vi "Vision Processing.vi"(8 "error in (no error)":errorcluster, 11 "Image Size":T2=enum."320x240") -> ()   [LabVIEW 2016]
uses:
  Program Files (x86)/National Instruments/LabVIEW 2016/examples/FRC/roboRIO/Vision/2017 Vision Example/Vision Support Code/Camera Types.ctl
  <vilib>/Rock Robotics/WPI/Camera/WPI_CameraImageSize.ctl
  <vilib>/Rock Robotics/WPI/Camera/WPI_CameraFrameRate.ctl
  <vilib>/Rock Robotics/WPI/Camera/WPI_CameraWhite Balance Values.ctl
  <vilib>/Rock Robotics/WPI/Camera/WPI_CameraExposure Values.ctl
  Robot Global Data.vi
  <vilib>/Rock Robotics/Network Tables/NT Write Number.vi
  <vilib>/vision/NI_Vision_Development_Module.lvlib
panel:
  in  "Frame Rate (fps)":T1=5
  in  "No vis code espos %":dbl format="%#_13g"
  out "error out":errorcluster
  in  "Size Limit %":dbl=0.02 format="%#_13g"
  in  "Ideal Target Height (in)":dbl=10.0
  out "loop ms":u32
  out "Calibration error":errorcluster
  in  "Display Original":bool
  in  "Display Mask":bool
  in  "Line Border":cluster{"Top":dbl, "Bottom":dbl}={"Top"=6.0, "Bottom"=1.0}
  in  "Use Calibration":bool
  out "Instructions:":string="Use Source to load image files from a directory, or use a USB or IP camera connected to your laptop. Use Camera Settings 1 and 2 to achieve a dark image with bright and colorful stripes.\nLED Color can encoded as HSL or related color modes. Calibrate to the same color as the strips being reflected to the camera.\nClick and draw a line in Original Image to auto-calibrate the LED Color. You may want to widen and tweak Sat and Val by hand.\nThe Annotate button affects drawing a rectangle around the stripes and labeling it with a distance in ft. Distance relies on knowing the Camera Type and lens calibration (it looks up the lens view angle).\n\nAdjust Score Cutoff to make the code more or less picky. If the color is not very unique, you may need to increase the number of particles considered. The diagram uses a Size Limit to ignore colored things that are too small. You may need to adjust it if you are targetting from far away.\n\nResults give you the distance to the target, the center and box in a normalized (-1 to 1) and pixel coordinates.\n\nBe sure to read about setting camera exposure and brightness to help simplify your image and acquire color saturated images.\n\nThere are lots of comments on the diagram to explain the code."
  in  "Color Mode":u16(ring)=3 items=["RGB", "HSL", "HSV", "HSI"]
  in  "Particles":dbl=5.0
  in  "Score Cutoff %":dbl=70.0
  in  "Camera Type":T3=enum."MS HD3000 640x480"
  out "Results":T4 {"Score" format="%#_3g"; "Pixels"."Rectangle"."Numeric 5" format="%#_3g"; "Pixels"."Rectangle"."Numeric 3" format="%#_3g"; "Pixels"."Rectangle"."Numeric 2" format="%#_3g"; "Pixels"."Rectangle"."Numeric" format="%#_3g"; "Normalized"."Rectangle"."Numeric 5" format="%#_2g"; "Normalized"."Rectangle"."Numeric 3" format="%#_2g"; "Normalized"."Rectangle"."Numeric 2" format="%#_2g"; "Normalized"."Rectangle"."Numeric" format="%#_2g"; "Normalized"."Center"."?" format="%#_3g"; "Normalized"."Center"."?" format="%#_3g"; "Distance (ft)" format="%#_3g"}
  out "Qualified Particles":i32
  in  "LED Color":T5={"Hue"={92.0569503435165, 129.13526899568942}, "Sat"={176.07142857142858, 255.0}, "Val"={40.53571428571429, 255.0}} {"Hue" scale=0.0..255.0 scale format="%#_3g"}
  out "Mask":T6(plugin-control)
  out "Original Image":T6(plugin-control)
  # "Legend:\n    Rectangle\n       Green - Good target, distance ft\n       Red - Bad target\n    Orange Text - Score in %"
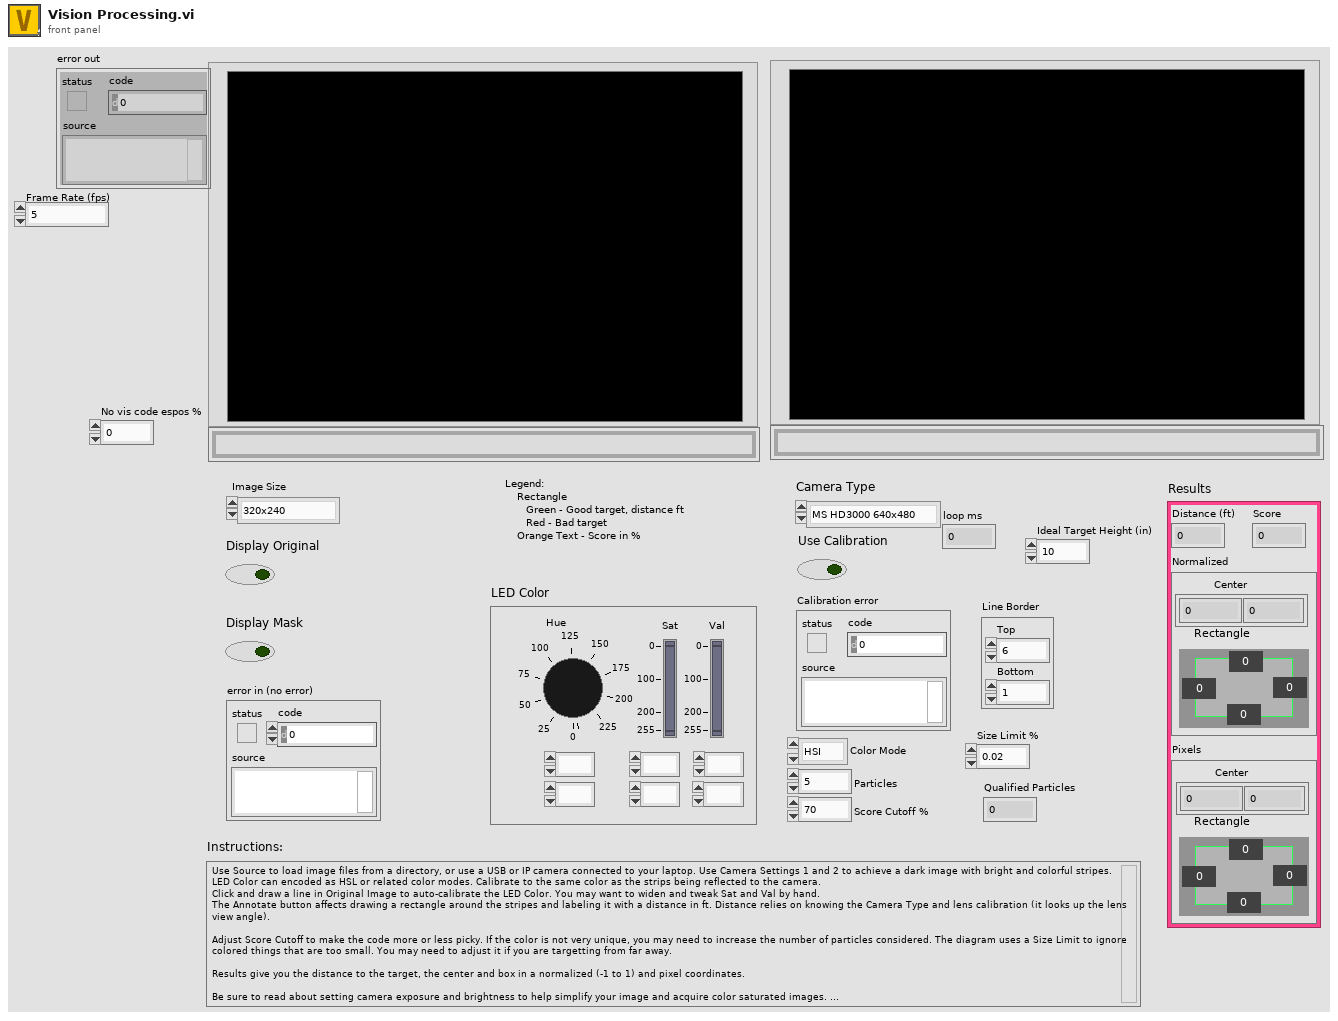
[diagram p1: front panel]
types:
  T1 = typedef "WPI_CameraFrameRate.ctl" = u32
  T2 = typedef "WPI_CameraImageSize.ctl" = enum16{"640x480", "320x240", "160x120", "Custom"}
  T3 = typedef "Camera Types.ctl" = enum16{"206", "1011", "1013", "MS HD3000 square", "MS HD3000 640x480"}
  T4 = cluster{"Distance (ft)":dbl, "Score":dbl, "Normalized":cluster{"Center":cluster{dbl, dbl}, "Rectangle":cluster{"Numeric":dbl, "Numeric 2":dbl, "Numeric 3":dbl, "Numeric 5":dbl}}, "Pixels":cluster{"Center":cluster{dbl, dbl}, "Rectangle":cluster{"Numeric":dbl, "Numeric 2":dbl, "Numeric 3":dbl, "Numeric 5":dbl}}}
  T5 = cluster{"Hue":cluster{dbl, dbl}, "Sat":cluster{dbl, dbl}, "Val":cluster{dbl, dbl}}
  T6 = typedef "IMAQ Image.ctl" = refnum<image>
  T7 = typedef "WPI_CameraWhite Balance Values.ctl" = enum16{"Auto", "Fixed indoor", "Fixed outdoor 1", "Fixed outdoor 2", "Fixed fluorescent 1", "Fixed fluorescent 2", "Hold current", "Custom"}
  T8 = typedef "Particle Parameters" = i32
  T9 = typedef "Image Type" = u32
  T10 = typedef "WPI_CameraDevRef.ctl" = cluster{"Camera Address":string, "CameraStatus":errorcluster}
  T11 = typedef "WPI_CameraExposure Values.ctl" = enum16{"Auto", "Flicker-free 50 Hz", "Flicker-free 60 Hz", "Hold current", "Custom"}
  T12 = cluster{"Left":dbl, "Top":dbl, "Right":dbl, "Bottom":dbl}
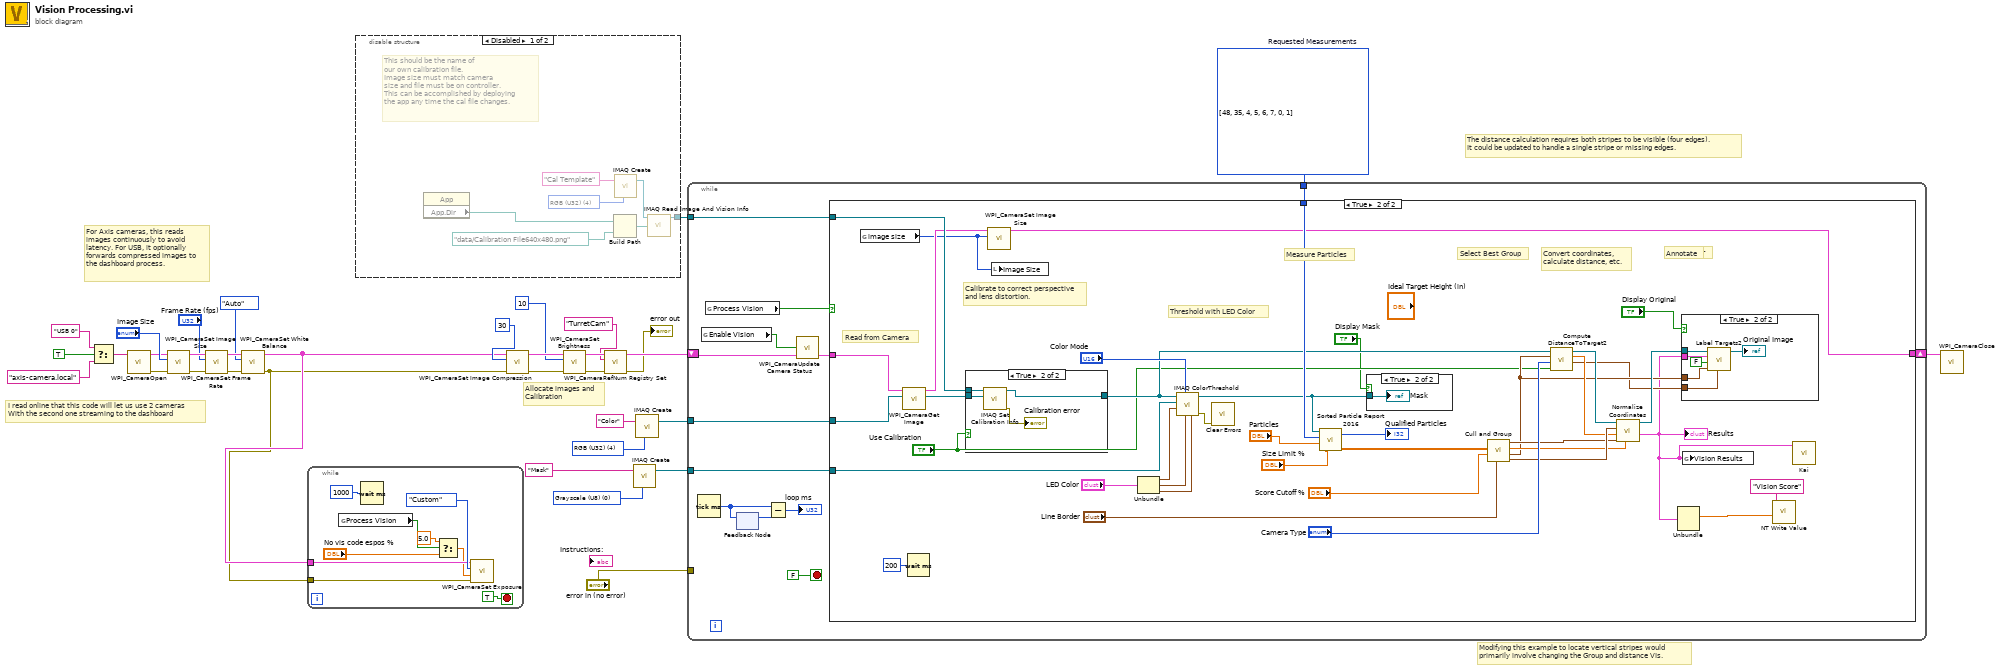
[diagram p0: block diagram]
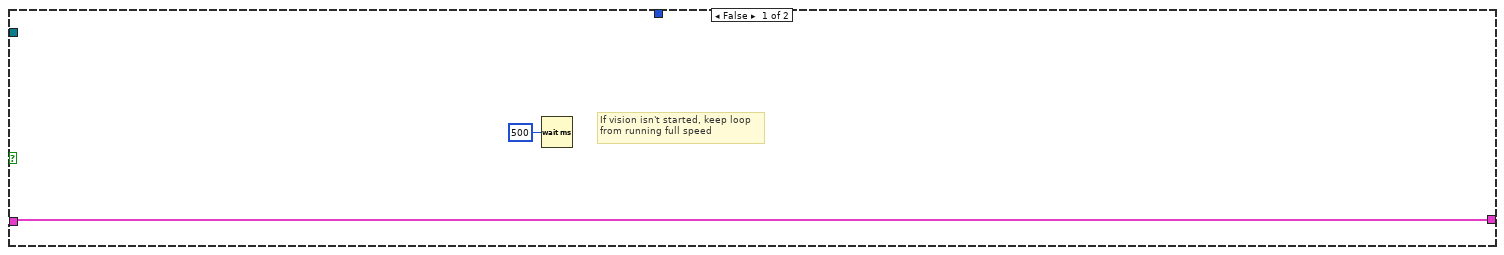
[diagram p3: hidden frame]
diagram:
  w29 = T8[] [48, 35, 4, 5, 6, 7, 0, 1] items=["Center of Mass X", "Center of Mass Y", "First Pixel X", "First Pixel Y", "Bounding Rect Left", "Bounding Rect Top", "Bounding Rect Right", "Bounding Rect Bottom", "Max Feret Diameter Start X", "Max Feret Diameter Start Y", "Max Feret Diameter End X", "Max Feret Diameter End Y", "Max Horiz. Segment Length Left", "Max Horiz. Segment Length Right", "Max Horiz. Segment Length Row", "-", "Bounding Rect Width", "Bounding Rect Height", "Bounding Rect Diagonal", "Perimeter", "Convex Hull Perimeter", "Holes' Perimeter", "Max Feret Diameter", "Equivalent Ellipse Major Axis", "Equivalent Ellipse Minor Axis", "Equivalent Ellipse Minor Axis (Feret)", "Equivalent Rect Long Side", "Equivalent Rect Short Side", "Equivalent Rect Diagonal", "Equivalent Rect Short Side (Feret)", "Average Horiz. Segment Length", "Average Vert. Segment Length", "Hydraulic Radius", "Waddel Disk Diameter", "-", "Area", "Holes' Area", "Particle & Holes' Area", "Convex Hull Area", "Image Area", "-", "Number of Holes", "Number of Horiz. Segments", "Number of Vert. Segments", "-", "Orientation", "Max Feret Diameter Orientation", "-", "% Area/Image Area", "% Area/(Particle & Holes' Area)", "Ratio of Equivalent Ellipse Axes", "Ratio of Equivalent Rect Sides", "-", "Elongation Factor", "Compactness Factor", "Heywood Circularity Factor", "Type Factor", "-", "Sum X", "Sum Y", "Sum XX", "Sum XY", "Sum YY", "Sum XXX", "Sum XXY", "Sum XYY", "Sum YYY", "-", "Moment of Inertia XX", "Moment of Inertia XY", "Moment of Inertia YY", "Moment of Inertia XXX", "Moment of Inertia XXY", "Moment of Inertia XYY", "Moment of Inertia YYY", "Norm. Moment of Inertia XX", "Norm. Moment of Inertia XY", "Norm. Moment of Inertia YY", "Norm. Moment of Inertia XXX", "Norm. Moment of Inertia XXY", "Norm. Moment of Inertia XYY", "Norm. Moment of Inertia YYY", "Hu Moment 1", "Hu Moment 2", "Hu Moment 3", "Hu Moment 4", "Hu Moment 5", "Hu Moment 6", "Hu Moment 7"]  # Requested Measurements
  w32 = T9 0 items=["Grayscale (U8)", "Grayscale (I16)", "Grayscale (SGL)", "Complex (CSG)", "RGB (U32)", "HSL (U32)", "RGB (U64)", "Grayscale (U16)"] ("Image Type")
  w33 = T9 4 items=["Grayscale (U8)", "Grayscale (I16)", "Grayscale (SGL)", "Complex (CSG)", "RGB (U32)", "HSL (U32)", "RGB (U64)", "Grayscale (U16)"] ("Image Type")
  # "I read online that this code will let us use 2 cameras\nWith the second one streaming to the dashboard"
  # "For Axis cameras, this reads\nimages continuously to avoid\nlatency. For USB, it optionally\nforwards compressed images to\nthe dashboard process."
  # "Modifying this example to locate vertical stripes would\nprimarily involve changing the Group and distance VIs."
  # "The distance calculation requires both stripes to be visible (four edges).\nIt could be updated to handle a single stripe or missing edges."
  # "Allocate images and\nCalibration"
  n1 = Select(t="USB 0" ("format string"), s=TRUE ("dot notation? (F)"), f="axis-camera.local" ("format string")) -> (s? t:f=w8:string)
  n2 = call <vilib>:"WPI_CameraOpen.vi"("Camera Address"=w8) -> ("error out"=w17:errorcluster, "CameraDevRef"=w18:T10)  [unwired: 2 in, 7 out]
  n3 = call <vilib>:"WPI_CameraSet Image Size.vi"("error in (no error)"=w17, "Image Size"="Image Size", "CameraDevRef"=w18) -> ("error out"=w16:errorcluster, "CameraDevRef Out"=w19:T10)  [unwired: 1 in, 6 out]
  n4 = call <vilib>:"WPI_CameraSet Frame Rate.vi"("error in (no error)"=w16, "Frame Rate (fps)"="Frame Rate (fps)", "CameraDevRef"=w19) -> ("error out"=w15:errorcluster, "CameraDevRef Out"=w20:T10)  [unwired: 7 out]
  n5 = call <vilib>:"WPI_CameraSet White Balance.vi"("error in (no error)"=w15, "White Balance"=WPI_CameraWhite_Balance_Values."Auto", "CameraDevRef"=w20) -> ("error out"=w1:errorcluster, "CameraDevRef Out"=w2:T10)  [unwired: 1 in, 6 out]
  n6 = while {
    tunnel: w2 -> [w42]
    tunnel: w1 -> [w41]
    stop <- TRUE stop-if-true
    n7 = global read "Robot Global Data.vi" "Process Vision"() -> (w38:bool)
    n8 = Wait (ms)(milliseconds to wait=u32 1000) -> ()  [unwired: 1 out]
    n9 = Select(t=5.0 ("Exposure (%)"), s=w38, f="No vis code espos %") -> (s? t:f=w35:dbl)
    n10 = call <vilib>:"WPI_CameraSet Exposure.vi"("error in (no error)"=w41, "Exposure (%)"=w35, "Exposure"=WPI_CameraExposure_Values."Custom", "CameraDevRef"=w42) -> ()  [unwired: 8 out]
  }
  n11 = disable-structure shown="Disabled" {
    disable-tunnel: [w47 _] -> w27
    frame Disabled {
      w50 = T9 4 items=["Grayscale (U8)", "Grayscale (I16)", "Grayscale (SGL)", "Complex (CSG)", "RGB (U32)", "HSL (U32)", "RGB (U64)", "Grayscale (U16)"] ("Image Type")
      # "This should be the name of \nour own calibration file.\nImage size must match camera\nsize and file must be on controller.\nThis can be accomplished by deploying\nthe app any time the cal file changes."
      n12 = property class="App"() -> ("App.Dir"=w44:path)  [unwired: 2 in, 2 out]
      n13 = Build Path(base path=w44, name or relative path=path "data/Calibration File640x480.png" ("Folder Location")) -> (appended path=w46:path)
      n14 = call "IMAQ Create"("Image Name"="Cal Template", "Image Type"=w50) -> ("New Image"=w48:T6)  [unwired: 2 in, 2 out]
      n15 = call "IMAQ Read Image And Vision Info"("File Path"=w46, "Image"=w48) -> ("Image Out"=w47:T6)  [unwired: 7 in, 2 out]
    }
    frame Enabled {
    }
  }
  n16 = call <vilib>:"WPI_CameraSet Image Compression.vi"("error in (no error)"=w1, "Compression"=30, "CameraDevRef"=w2) -> ("error out"=w14:errorcluster, "CameraDevRef Out"=w21:T10)  [unwired: 7 out]
  n17 = call <vilib>:"WPI_CameraSet Brightness.vi"("error in (no error)"=w14, "Brightness"=10, "CameraDevRef"=w21) -> ("error out"=w13:errorcluster, "CameraDevRef Out"=w26:T10)  [unwired: 7 out]
  n18 = call <vilib>:"WPI_CameraRefNum Registry Set.vi"("error in (no error)"=w13, "refnum name"="TurretCam", "CameraDevRef"=w26) -> ("error out"=→"error out":errorcluster, "CameraDevRef"=w7:T10)  [unwired: 1 in, 6 out]
  n19 = call "IMAQ Create"("Image Name"="Mask", "Image Type"=w32) -> ("New Image"=w30:T6)  [unwired: 2 in, 2 out]
  n20 = call "IMAQ Create"("Image Name"="Color", "Image Type"=w33) -> ("New Image"=w28:T6)  [unwired: 2 in, 2 out]
  n21 = while {
    tunnel: w28 -> [w59]
    tunnel: w30 -> [w62]
    tunnel: w29 -> [w61]
    tunnel: w27 -> [w60]
    shift-right: [w58] -> w6
    shift-left: w7 -> [w57]
    tunnel: "error in (no error)" -> [_]
    stop <- FALSE stop-if-true
    n22 = Tick Count (ms)() -> (millisecond timer value=w53:u32)
    n23 = global read "Robot Global Data.vi" "Enable Vision"() -> (w51:bool)
    n24 = global read "Robot Global Data.vi" "Process Vision"() -> (w55:bool)
    n25 = feedback-in #1(w53) -> ()
    n26 = feedback #1() -> (w54:u32)  [unwired: 1 in]
    n27 = Subtract(x=w53, y=w54) -> (x-y=→"loop ms":u32)
    n28 = call <vilib>:"WPI_CameraUpdate Camera Status.vi"("CameraDevRef In"=w57, "Enable Vision"=w51) -> ("CameraDevRef Out"=w56:T10)  [unwired: 3 in]
    n29 = case shown="True" w55 {
      tunnel: w62 -> [_ w104]
      tunnel: w61 -> [_ w100]
      tunnel: w60 -> [_ w80]
      tunnel: w56 -> [w65 w77]
      tunnel: w59 -> [_ w76]
      tunnel: [w65 w71] -> w58
      frame False {
        # "If vision isn't started, keep loop\nfrom running full speed"
        n30 = Wait (ms)(milliseconds to wait=u32 500) -> ()  [unwired: 1 out]
      }
      frame True {
        # "Write to NT"
        # "Read from Camera"
        # "Calibrate to correct perspective\nand lens distortion."
        # "Measure Particles"
        # "Convert coordinates,\ncalculate distance, etc."
        # "Annotate"
        # "Select Best Group"
        # "Threshold with LED Color"
        n31 = global read "Robot Global Data.vi" "image size"() -> (w70:T2)
        n32 = call <vilib>:"WPI_CameraGet Image.vi"("Image"=w76, "CameraDevRef"=w77) -> ("Image Out"=w75:T6, "CameraDevRef Out"=w72:T10)  [unwired: 7 in, 1 out]
        n33 = Wait (ms)(milliseconds to wait=u32 200) -> ()  [unwired: 1 out]
        n34 = case shown="True" "Use Calibration" {
          tunnel: [w112 w116] -> w81
          tunnel: w75 -> [w112 w115]
          tunnel: w80 -> [_ w114]
          frame False {
          }
          frame True {
            n35 = call "IMAQ Set Calibration Info"("Image Dst"=w115, "Image Src"=w114) -> ("error out"=→"Calibration error":errorcluster, "Calibrated Image"=w116:T6)  [unwired: 8 in]
          }
        }
        n36 = call <vilib>:"WPI_CameraSet Image Size.vi"("Image Size"=w70, "CameraDevRef"=w72) -> ("CameraDevRef Out"=w71:T10)  [unwired: 2 in, 7 out]
        n37 = local write "Image Size"(w70) -> ()
        n38 = Unbundle("LED Color") -> ("Hue"=w103:cluster{dbl, dbl}, "Sat"=w102:cluster{dbl, dbl}, "Val"=w101:cluster{dbl, dbl})
        n39 = call "IMAQ ColorThreshold"("Blue or Luma or Val or Inten Range"=w101, "Green or Sat Range"=w102, "Color Mode"="Color Mode", "Red or Hue Range"=w103, "Image Dst"=w104, "Image Src"=w81) -> ("error out"=w97:errorcluster, "Image Dst Out"=w93:T6)  [unwired: 4 in]
        n40 = call <vilib>:"Clear Errors.vi"("error in (no error)"=w97) -> ()  [unwired: 5 in, 2 out]
        n41 = call "Sorted Particle Report 2016.vi"("Min Area Size %"="Size Limit %", "Particle Count Limit"="Particles", "Pixel Measurements"=w100, "Image in"=w93) -> ("Sorted Data"=w95:dbl[][], "Particles"=→"Qualified Particles":i32)
        n42 = case shown="True" "Display Mask" {
          tunnel: w93 -> [_ w111]
          frame False {
          }
          frame True {
            "Mask" <- w111
          }
        }
        n43 = call "Cull and Group.vi"("Line Border"="Line Border", "Score Cutoff"="Score Cutoff %", "Sorted Data"=w95) -> ("Rect"=w91:T12, "Line"=w83:T12, "Score"=w86:dbl, "Center"=w87:cluster{"X":dbl, "Y":dbl})  [unwired: 5 in]
        n44 = call "Compute DistanceToTarget2.vi"("Calibrated"="Use Calibration", "Camera Type"="Camera Type", "Line"=w83, "Image Src"=w81) -> ("Edges"=w82:cluster{"X":sgl, "Y":sgl}[], "Distance (ft)"=w90:dbl, "Image Dst Out"=w89:T6)  [unwired: 5 in]
        n45 = call "Normalize Coordinates.vi"("Score"=w86, "Center"=w87, "Distance"=w90, "Bounding box"=w91, "Image in"=w89) -> ("Results"=w67:T4, "Image out"=w88:T6)  [unwired: 5 in]
        "Results" <- w67
        n46 = Unbundle(w67) -> ("Score"=w69:dbl)  [unwired: 3 out]
        n47 = case shown="True" "Display Original" {
          tunnel: w88 -> [_ w109]
          tunnel: w67 -> [_ w108]
          tunnel: w83 -> [_ w107]
          tunnel: w82 -> [_ w106]
          frame False {
          }
          frame True {
            n48 = call "Label Targets2.vi"("Edges"=w106, "Line"=w107, "Annotate"=FALSE, "Results"=w108, "Image in"=w109) -> ("Image out"=→"Original Image":T6)  [unwired: 6 in]
          }
        }
        n49 = global write "Robot Global Data.vi" "Vision Results"(w67) -> ()
        n50 = call-poly <vilib>:"NT Write Value.vi"("Numeric"=w69, "Name"="Vision Score") -> ()  [unwired: 9 in, 1 out]
        n51 = call "Kai.vi"("Vision Results"=w67) -> ()  [unwired: 11 in]
      }
    }
  }
  n52 = call <vilib>:"WPI_CameraClose.vi"("CameraDevRef"=w6) -> ()  [unwired: 1 in, 10 out]
